vi "Config Spark Max SLOT Close Loop HW Get Set.vi"(4 "PIDF Slot (0)":i32, 6 "Get(f) Set(t)":bool, 7 "SparkMax Slot CL":T1={"Gains"={"P"=0.1, "I"=0.0, "D"=0.0, "F"=0.0}, "I Zone"=1.0, "Peak Out -1 0 1"={"High"=0.0, "Low"=0.0}, "Max I Accu"=0.0} {"Gains"."F" format="%#.8f"; "Gains"."D" format="%#.8f"; "Gains"."I" format="%#.8f"; "Gains"."P" format="%#.8f"; "Peak Out -1 0 1"."Low" format="%#.8f"; "Peak Out -1 0 1"."High" format="%#.8f"}, 8 "Error":errorcluster, 11 "Drive Refs":T4) -> (0 "Error Out":errorcluster, 3 "Drive Refs Out":T4, 5 "SparkMax Slot CL Out":T1={"Gains"={"P"=0.1, "I"=0.0, "D"=0.0, "F"=0.0}, "I Zone"=1.0, "Peak Out -1 0 1"={"High"=0.0, "Low"=0.0}, "Max I Accu"=0.0} {"Gains"."F" format="%#.8f"; "Gains"."D" format="%#.8f"; "Gains"."I" format="%#.8f"; "Gains"."P" format="%#.8f"; "Peak Out -1 0 1"."Low" format="%#.8f"; "Peak Out -1 0 1"."High" format="%#.8f"})   [LabVIEW 2023, in "Swerve-SteerSRX-DriveSpark-AbsAnalog_ACT.lvlib"]
uses:
  Swerve-SteerSRX-DriveSpark-AbsAnalog_ACT.lvlib
  <vilib>/Rock Robotics/WPI/MotorControl/WPI_MotorControlDeviceRef.ctl
  <vilib>/Rock Robotics/WPI/MotorControl/WPI_MotorControlType.ctl
  <vilib>/Rock Robotics/SystemInterfaces/DIO/FPGA_DIOPWMChannel.ctl
  <vilib>/Rock Robotics/WPI/PWM/WPI_PWMDeadband.ctl
  <vilib>/Rock Robotics/SystemInterfaces/DIO/FPGA_DIOChannel.ctl
  Shared Code/TypeDefs/Cluster_Spark MAX Config_SLOT PID Config.ctl
  Shared Code/TypeDefs/Cluster_PID Gains.ctl
  Shared Code/TypeDefs/Cluster_High-Low.ctl
  Shared Code/TypeDefs/Cluster_SRX SLOT PID Config.ctl
  <vilib>/Utility/error.llb/Trim Whitespace One-Sided.vi
  <vilib>/Utility/Data Type/NI_Data Type.lvlib
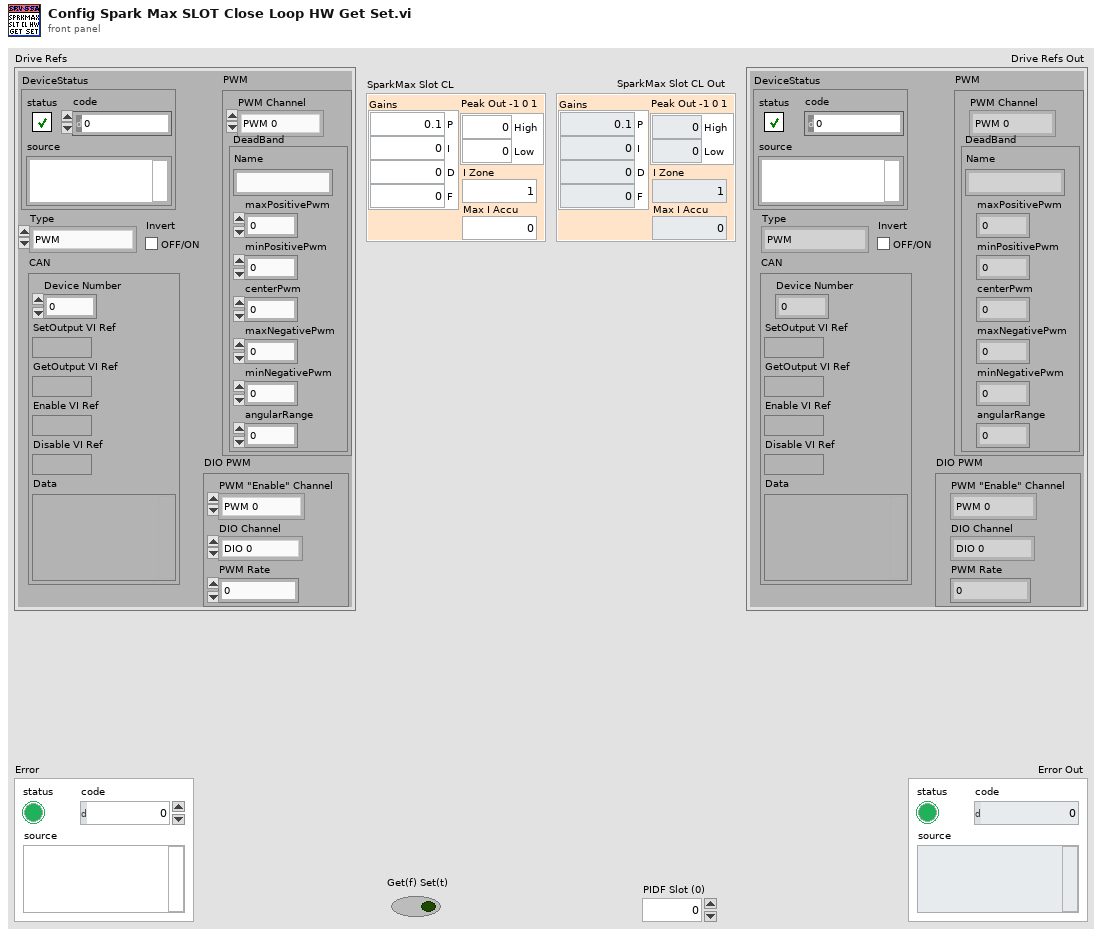
[diagram p1: front panel]
types:
  T1 = typedef "Cluster_Spark MAX Config_SLOT PID Config.ctl" = cluster{"Gains":T2, "I Zone":dbl, "Peak Out -1 0 1":T3, "Max I Accu":dbl}
  T2 = typedef "Cluster_PID Gains.ctl" = cluster{"P":dbl, "I":dbl, "D":dbl, "F":dbl}
  T3 = typedef "Cluster_High-Low.ctl" = cluster{"High":dbl, "Low":dbl}
  T4 = typedef "WPI_MotorControlDeviceRef.ctl" = cluster{"DeviceStatus":errorcluster, "Type":T5, "PWM":cluster{"PWM Channel":T6, "DeadBand":T7}, "CAN":cluster{"Device Number":u8, "SetOutput VI Ref":variant, "GetOutput VI Ref":variant, "Enable VI Ref":variant, "Disable VI Ref":variant, "Data":variant}, "Invert":bool, "DIO PWM":cluster{"PWM \"Enable\" Channel":T6, "DIOChannel":T8, "PWM Rate":dbl}}
  T5 = typedef "WPI_MotorControlType.ctl" = enum16{"PWM", "CAN", "DIO PWM"}
  T6 = typedef "FPGA_DIOPWMChannel.ctl" = enum8{"PWM 0", "PWM 1", "PWM 2", "PWM 3", "PWM 4", "PWM 5", "PWM 6", "PWM 7", "PWM 8", "PWM 9", "PWM MXP 0", "PWM MXP 1", "PWM MXP 2", "PWM MXP 3", "PWM MXP 4", "PWM MXP 5", "PWM MXP 6", "PWM MXP 7", "PWM MXP 8", "PWM MXP 9", "Invalid"}
  T7 = typedef "WPI_PWMDeadband.ctl" = cluster{"Name":string, "maxPositivePwm":i32, "minPositivePwm":i32, "centerPwm":i32, "maxNegativePwm":i32, "minNegativePwm":i32, "angularRange":u16}
  T8 = typedef "FPGA_DIOChannel.ctl" = enum8{"DIO 0", "DIO 1", "DIO 2", "DIO 3", "DIO 4", "DIO 5", "DIO 6", "DIO 7", "DIO 8", "DIO 9", "DIO MXP 0", "DIO MXP 1", "DIO MXP 2", "DIO MXP 3", "DIO MXP 4", "DIO MXP 5", "DIO MXP 6", "DIO MXP 7", "DIO MXP 8", "DIO MXP 9", "DIO MXP 10", "DIO MXP 11", "DIO MXP 12", "DIO MXP 13", "DIO MXP 14", "DIO MXP 15", "SPI Port CS1", "SPI Port CS2", "SPI Port CS3", "SPI Port MISO", "SPI Port MOSI", "Invalid"}
  T9 = typedef "Cluster_SRX SLOT PID Config.ctl" = cluster{"Gains":T2, "Error Allowed":dbl, "I Zone":dbl, "Peak Out 0-1":dbl, "Max I Accu":dbl}
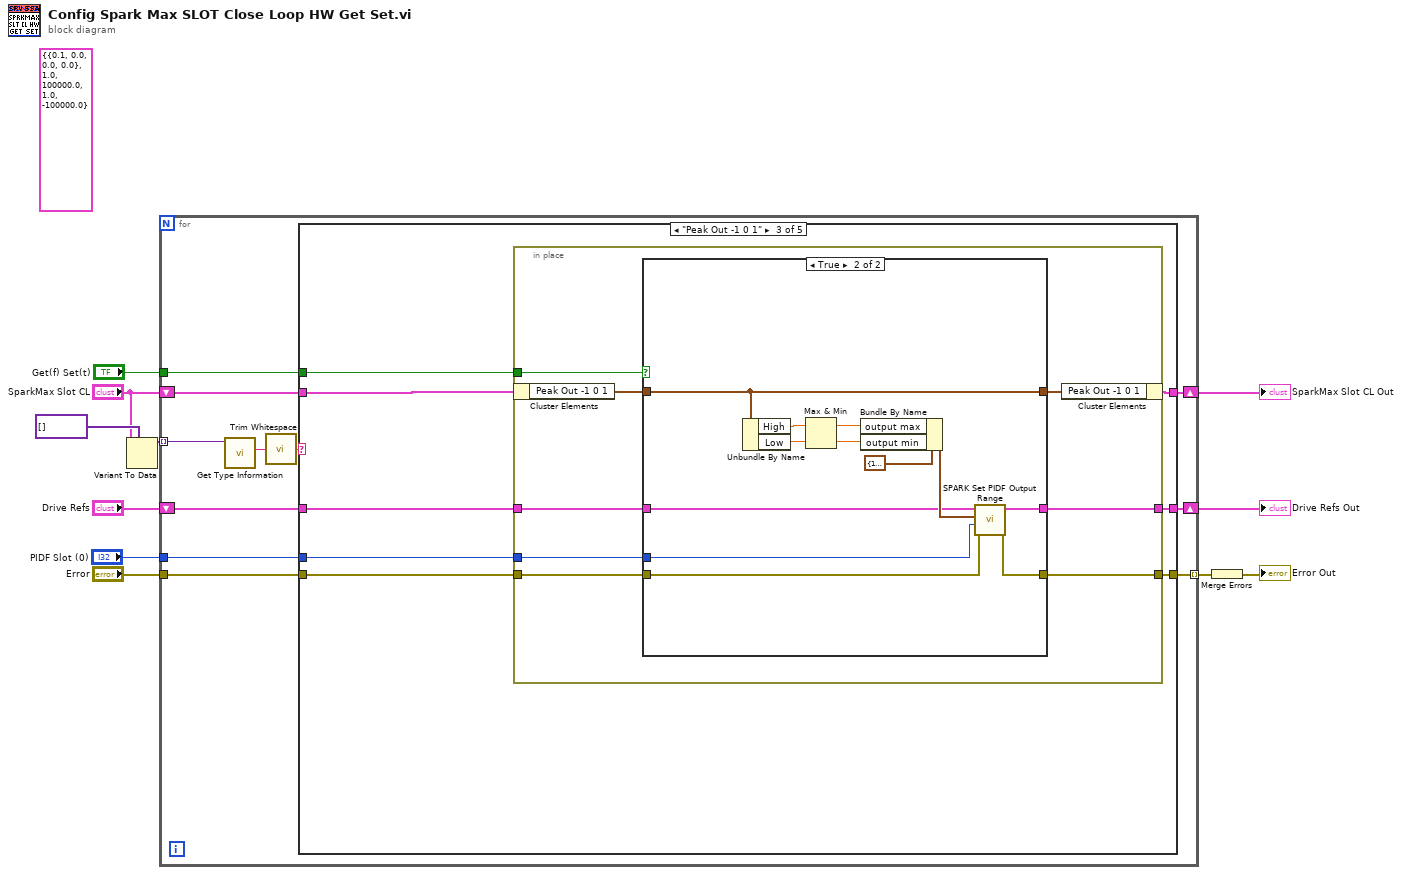
[diagram p0: block diagram]
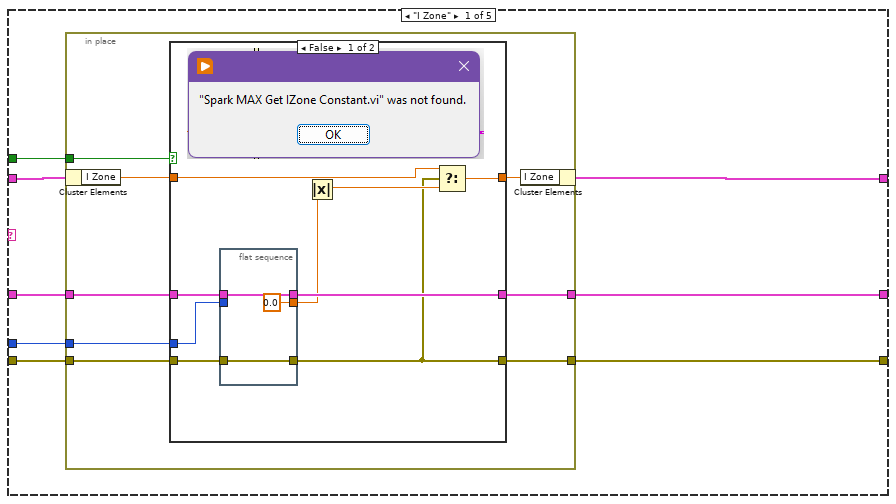
[diagram p2: hidden frame]
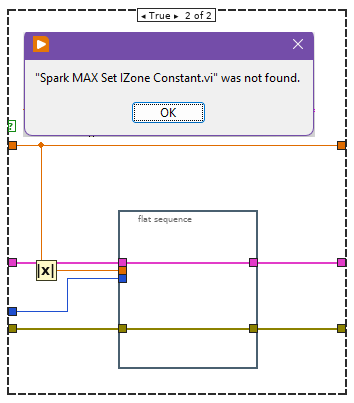
[diagram p3: hidden frame]
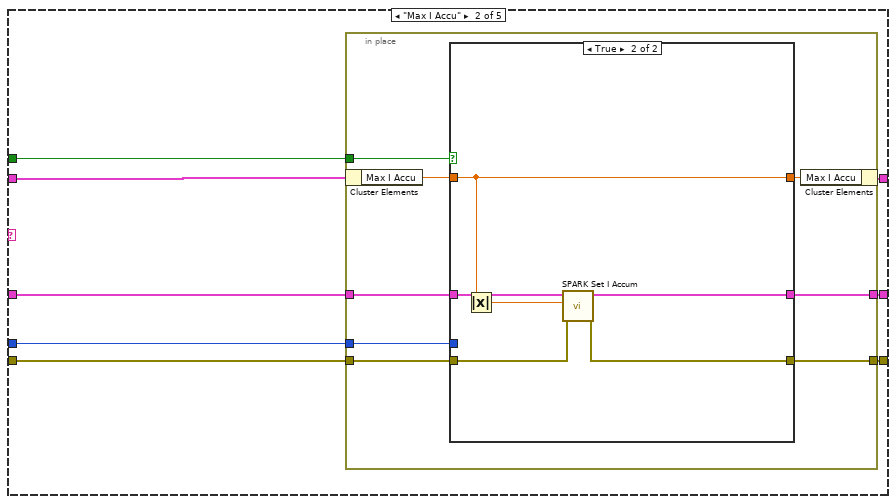
[diagram p4: hidden frame]
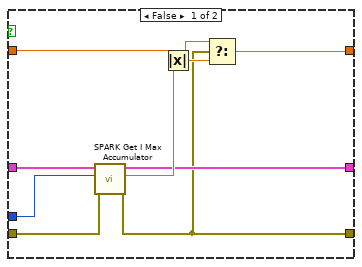
[diagram p5: hidden frame]
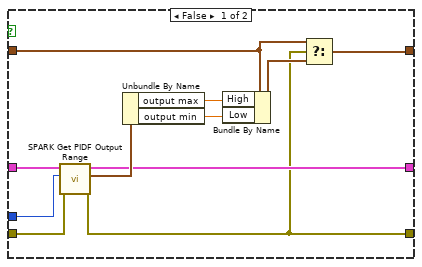
[diagram p6: hidden frame]
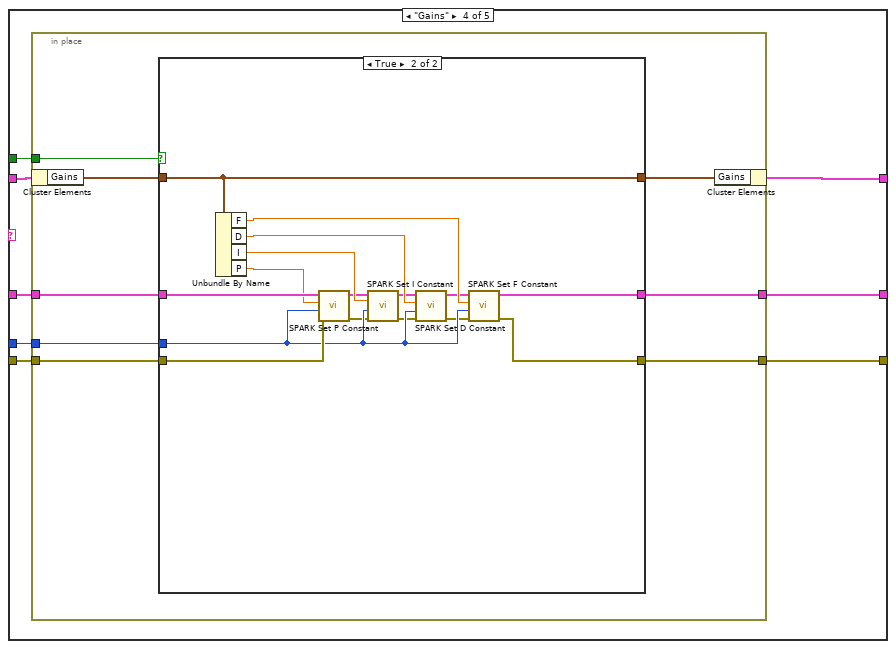
[diagram p7: hidden frame]
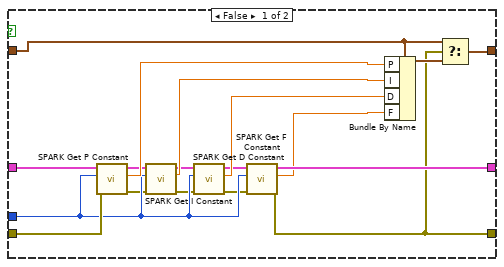
[diagram p8: hidden frame]
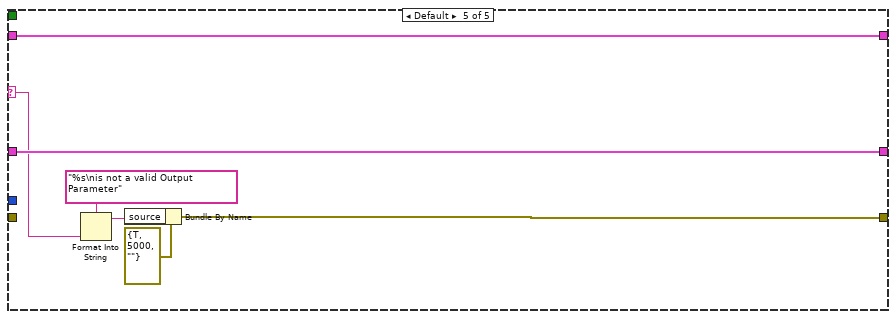
[diagram p9: hidden frame]
diagram:
  (unwired) T9 {"Gains"={"P"=0.1, "I"=0.0, "D"=0.0, "F"=0.0}, "Error Allowed"=1.0, "I Zone"=100000.0, "Peak Out 0-1"=1.0, "Max I Accu"=-100000.0} ("SparkMax Output")
  n1 = Variant To Data(type=variant[] [], Variant="SparkMax Slot CL") -> (data=w6:variant[])  [unwired: 1 in, 1 out]
  n2 = for {
    shift-right: [w13] -> w11
    shift-left: "SparkMax Slot CL" -> [w19]
    shift-right: [w14] -> w9
    shift-left: "Drive Refs" -> [w18]
    tunnel: "Get(f) Set(t)" -> [w17]
    tunnel: w6 -> [w21] mode=indexing
    tunnel: "Error" -> [w16]
    tunnel: [w15] -> w3 mode=indexing
    tunnel: "PIDF Slot (0)" -> [w12]
    n3 = call <vilib>:"Get Type Information.vi"("variant"=w21) -> ("name"=w22:string)  [unwired: 6 in, 4 out]
    n4 = call <vilib>:"Trim Whitespace.vi"("string"=w22) -> ("trimmed string"=w20:string)  [unwired: 1 in]
    n5 = case shown="\"Peak Out -1 0 1\"" w20 {
      selector: w20 -> [_ _ _ _ w184]
      tunnel: w19 -> [w30 w67 w98 w137 w186]
      tunnel: w18 -> [w26 w63 w94 w133 w185]
      tunnel: w17 -> [w29 w66 w97 w136 _]
      tunnel: w16 -> [w28 w65 w96 w135 _]
      tunnel: [w27 w64 w95 w134 w182] -> w15
      tunnel: [w25 w62 w93 w132 w185] -> w14
      tunnel: [w24 w61 w92 w131 w186] -> w13
      tunnel: w12 -> [w23 w60 w91 w130 _]
      frame "I Zone" {
        n6 = in-place {
          in-place-border: w29 -> [w38]
          in-place-border: w28 -> [w36]
          in-place-border: [w35] -> w27
          in-place-border: w26 -> [w34]
          in-place-border: [w33] -> w25
          in-place-border: w23 -> [w31]
          n7 = in-place-cluster #1(w30) -> ("I Zone"=w37:dbl)
          n8 = case shown="False" w38 {
            tunnel: w37 -> [w46 w57]
            tunnel: w36 -> [w40 w52]
            tunnel: [w39 w51] -> w35
            tunnel: w34 -> [w43 w56]
            tunnel: [w42 w55] -> w33
            tunnel: [w47 w57] -> w32
            tunnel: w31 -> [w44 w53]
            frame False {
              n9 = flat-sequence {
                tunnel: w44 -> [_]
                tunnel: w43 -> [w50]
                tunnel: [w50] -> w42
                tunnel: [0.0 ("IZone")] -> w41
                tunnel: w40 -> [w49]
                tunnel: [w49] -> w39
                frame #0 {
                }
              }
              n10 = Absolute Value(x=w41) -> (abs(x)=w45:dbl)
              n11 = Select(t=w46, s=w39, f=w45) -> (s? t:f=w47:dbl)
            }
            frame True {
              n12 = Absolute Value(x=w57) -> (abs(x)=w54:dbl)
              n13 = flat-sequence {
                tunnel: w56 -> [w58]
                tunnel: [w58] -> w55
                tunnel: w54 -> [_]
                tunnel: w53 -> [_]
                tunnel: w52 -> [w59]
                tunnel: [w59] -> w51
                frame #0 {
                }
              }
            }
          }
          n14 = in-place-cluster #1("I Zone"=w32) -> (w24:T1)
        }
      }
      frame "Max I Accu" {
        n15 = in-place {
          in-place-border: w66 -> [w75]
          in-place-border: w65 -> [w73]
          in-place-border: [w72] -> w64
          in-place-border: w63 -> [w71]
          in-place-border: [w70] -> w62
          in-place-border: w60 -> [w68]
          n16 = in-place-cluster #2(w67) -> ("Max I Accu"=w74:dbl)
          n17 = case shown="True" w75 {
            tunnel: w74 -> [w83 w90]
            tunnel: w73 -> [w77 w86]
            tunnel: [w76 w85] -> w72
            tunnel: w71 -> [w79 w89]
            tunnel: [w80 w88] -> w70
            tunnel: [w84 w90] -> w69
            tunnel: w68 -> [w78 _]
            frame False {
              n18 = call <vilib>:"SPARK Get I Max Accumulator.vi"("error in (no error)"=w77, "PIDF Slot (0)"=w78, "MotorControlDeviceRef in"=w79) -> ("error out"=w76:errorcluster, "Max Accumulator"=w81:dbl, "MotorControlDeviceRef out"=w80:T4)  [unwired: 6 in]
              n19 = Absolute Value(x=w81) -> (abs(x)=w82:dbl)
              n20 = Select(t=w83, s=w76, f=w82) -> (s? t:f=w84:dbl)
            }
            frame True {
              n21 = Absolute Value(x=w90) -> (abs(x)=w87:dbl)
              n22 = call <vilib>:"SPARK Set I Accum.vi"("error in"=w86, "I Accum"=w87, "MotorControlDeviceRef"=w89) -> ("error out"=w85:errorcluster, "MotorControlDeviceRef"=w88:T4)  [unwired: 7 in]
            }
          }
          n23 = in-place-cluster #2("Max I Accu"=w69) -> (w61:T1)
        }
      }
      frame "Peak Out -1 0 1" {
        n24 = in-place {
          in-place-border: w97 -> [w106]
          in-place-border: w96 -> [w104]
          in-place-border: [w103] -> w95
          in-place-border: w94 -> [w102]
          in-place-border: [w101] -> w93
          in-place-border: w91 -> [w99]
          n25 = in-place-cluster #3(w98) -> ("Peak Out -1 0 1"=w105:T3)
          n26 = case shown="True" w106 {
            tunnel: w105 -> [w116 w128]
            tunnel: w104 -> [w108 w120]
            tunnel: [w107 w118] -> w103
            tunnel: w102 -> [w110 w122]
            tunnel: [w111 w121] -> w101
            tunnel: [w117 w128] -> w100
            tunnel: w99 -> [w109 w119]
            frame False {
              n27 = call <vilib>:"SPARK Get PIDF Output Range.vi"("error in (no error)"=w108, "PIDF Slot (0)"=w109, "MotorControlDeviceRef in"=w110) -> ("error out"=w107:errorcluster, "output range"=w112:cluster{"output max":dbl, "output min":dbl}, "MotorControlDeviceRef out"=w111:T4)  [unwired: 6 in]
              n28 = Unbundle By Name(w112) -> ("output max"=w114:dbl, "output min"=w113:dbl)
              n29 = Bundle By Name(cluster=w116, "High"=w114, "Low"=w113) -> (w115:T3)
              n30 = Select(t=w116, s=w107, f=w115) -> (s? t:f=w117:T3)
            }
            frame True {
              n31 = Unbundle By Name(w128) -> ("High"=w127:dbl, "Low"=w125:dbl)
              n32 = Max & Min(x=w127, y=w125) -> (max(x,y)=w126:dbl, min(x,y)=w124:dbl)
              n33 = Bundle By Name(cluster=cluster{"output max":dbl, "output min":dbl} {"output max"=1.0, "output min"=-1.0} ("output range"), "output max"=w126, "output min"=w124) -> (w123:cluster{"output max":dbl, "output min":dbl})
              n34 = call <vilib>:"SPARK Set PIDF Output Range.vi"("error in"=w120, "PIDF Slot (0)"=w119, "output range"=w123, "MotorControlDeviceRef"=w122) -> ("error out"=w118:errorcluster, "MotorControlDeviceRef"=w121:T4)  [unwired: 6 in]
            }
          }
          n35 = in-place-cluster #3("Peak Out -1 0 1"=w100) -> (w92:T1)
        }
      }
      frame "Gains" {
        n36 = in-place {
          in-place-border: w136 -> [w145]
          in-place-border: w135 -> [w143]
          in-place-border: [w142] -> w134
          in-place-border: w133 -> [w141]
          in-place-border: [w140] -> w132
          in-place-border: w130 -> [w138]
          n37 = in-place-cluster #4(w137) -> ("Gains"=w144:T2)
          n38 = case shown="True" w145 {
            tunnel: w144 -> [w146 w175]
            tunnel: w143 -> [w158 w176]
            tunnel: [w159 w177] -> w142
            tunnel: w141 -> [w161 w179]
            tunnel: [w160 w178] -> w140
            tunnel: [w163 w175] -> w139
            tunnel: w138 -> [w153 w174]
            frame False {
              n39 = call <vilib>:"SPARK Get P Constant.vi"("error in (no error)"=w158, "PIDF Slot (0)"=w153, "MotorControlDeviceRef in"=w161) -> ("error out"=w149:errorcluster, "kP"=w157:dbl, "MotorControlDeviceRef out"=w152:T4)  [unwired: 6 in]
              n40 = call <vilib>:"SPARK Get I Constant.vi"("error in (no error)"=w149, "PIDF Slot (0)"=w153, "MotorControlDeviceRef in"=w152) -> ("error out"=w148:errorcluster, "kI"=w156:dbl, "MotorControlDeviceRef out"=w151:T4)  [unwired: 6 in]
              n41 = call <vilib>:"SPARK Get D Constant.vi"("error in (no error)"=w148, "PIDF Slot (0)"=w153, "MotorControlDeviceRef in"=w151) -> ("error out"=w147:errorcluster, "kD"=w155:dbl, "MotorControlDeviceRef out"=w150:T4)  [unwired: 6 in]
              n42 = call <vilib>:"SPARK Get F Constant.vi"("error in (no error)"=w147, "PIDF Slot (0)"=w153, "MotorControlDeviceRef in"=w150) -> ("error out"=w159:errorcluster, "kF"=w154:dbl, "MotorControlDeviceRef out"=w160:T4)  [unwired: 6 in]
              n43 = Bundle By Name(cluster=w146, "P"=w157, "I"=w156, "D"=w155, "F"=w154) -> (w162:T2)
              n44 = Select(t=w146, s=w159, f=w162) -> (s? t:f=w163:T2)
            }
            frame True {
              n45 = Unbundle By Name(w175) -> ("F"=w170:dbl, "D"=w171:dbl, "I"=w172:dbl, "P"=w173:dbl)
              n46 = call <vilib>:"SPARK Set P Constant.vi"("error in"=w176, "PIDF Slot"=w174, "kP"=w173, "MotorControlDeviceRef"=w179) -> ("error out"=w166:errorcluster, "MotorControlDeviceRef"=w169:T4)  [unwired: 6 in]
              n47 = call <vilib>:"SPARK Set I Constant.vi"("error in"=w166, "PIDF Slot"=w174, "kI"=w172, "MotorControlDeviceRef"=w169) -> ("error out"=w165:errorcluster, "MotorControlDeviceRef"=w168:T4)  [unwired: 6 in]
              n48 = call <vilib>:"SPARK Set D Constant.vi"("error in"=w165, "PIDF Slot"=w174, "kD"=w171, "MotorControlDeviceRef"=w168) -> ("error out"=w164:errorcluster, "MotorControlDeviceRef"=w167:T4)  [unwired: 6 in]
              n49 = call <vilib>:"SPARK Set F Constant.vi"("error in"=w164, "PIDF Slot"=w174, "kF"=w170, "MotorControlDeviceRef"=w167) -> ("error out"=w177:errorcluster, "MotorControlDeviceRef"=w178:T4)  [unwired: 6 in]
            }
          }
          n50 = in-place-cluster #4("Gains"=w139) -> (w131:T1)
        }
      }
      frame Default {
        n51 = Format Into String(format string="%s\nis not a valid Output Parameter", w184) -> (resulting string=w180:string)  [unwired: 2 in, 1 out]
        n52 = Bundle By Name(cluster=errorcluster {"status"=TRUE, "code"=5000, "source"=""} ("error out"), "source"=w180) -> (w182:errorcluster)
      }
    }
  }
  "Drive Refs Out" <- w9
  "SparkMax Slot CL Out" <- w11
  n53 = Merge Errors(w3) -> (→"Error Out":errorcluster)
